vi "DynamixelConfigure.vi"() -> ()   [LabVIEW 2013]
doc: "Set the Dynamixels to the settings we want. Should only need to be run one per group of Dynamixels - they're supposed to remember their settings.\n\nElizabeth Mahon, 4-7-2014"
uses:
  <instrlib>/Dynamixel Motor/Public/Motor Operation/Low Level/Baud Setting.ctl
  <instrlib>/Dynamixel Motor/Dynamixel Motor.lvlib
panel:
  out "Found right # of motors?":bool
  in  "# of motors":i32=3
  in  "VISA resource name":refnum<visa-resource-name>
  # "SET THESE BEFORE RUNNING!"
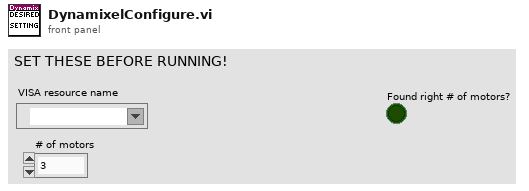
[diagram p1: front panel]
types:
  T1 = typedef "Dynamixel Motor.lvlib/Baud Setting.ctl" = u8
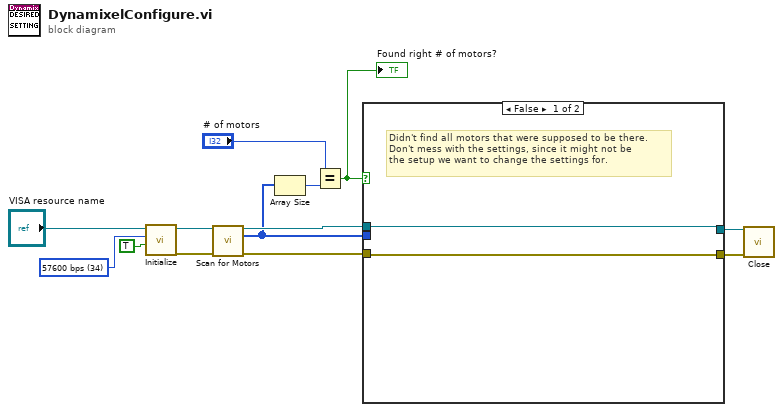
[diagram p0: block diagram]
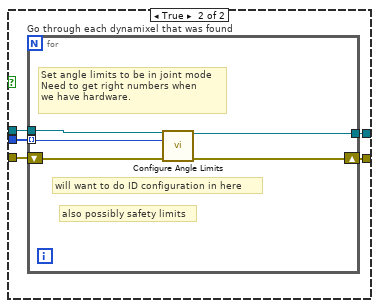
[diagram p2: hidden frame]
diagram:
  w12 = T1 34 items=["1,000,000 bps"=1, "500,000 bps"=3, "400,000 bps"=4, "250,000 bps"=7, "200,000 bps"=9, "115200 bps"=16, "57600 bps"=34, "19200 bps"=103, "9600 bps"=207] ("Baud rate (57600 bps)")
  n1 = call <instrlib>:"Initialize.vi"("Force Baud Rate (True)"=TRUE, "Baud rate (57600 bps)"=w12, "VISA resource name"="VISA resource name") -> ("error out"=w9:errorcluster, "VISA resource name out"=w10:refnum<visa-resource-name>)  [unwired: 7 in]
  n2 = call <instrlib>:"Scan for Motors.vi"("VISA resource name"=w10, "error in (no error)"=w9) -> ("VISA resource name out"=w8:refnum<visa-resource-name>, "Motors IDs Found"=w4:u8[], "error out"=w6:errorcluster)  [unwired: 11 in]
  n3 = Array Size(array=w4) -> (size(s)=w3:i32)
  n4 = Equal?(x="# of motors", y=w3) -> (x = y?=w1:bool)
  "Found right # of motors?" <- w1
  n5 = case shown="False" w1 {
    tunnel: w4 -> [_ w20]
    tunnel: w8 -> [w15 w19]
    tunnel: [w15 w18] -> w7
    tunnel: w6 -> [w14 w17]
    tunnel: [w14 w16] -> w5
    frame False {
      # "Didn't find all motors that were supposed to be there.\nDon't mess with the settings, since it might not be\nthe setup we want to change the settings for."
    }
    frame True {
      n6 = for "Go through each dynamixel that was found" {
        tunnel: w20 -> [w24] mode=indexing
        tunnel: w19 -> [w25]
        tunnel: [w23] -> w18
        shift-right: [w22] -> w16
        shift-left: w17 -> [w21]
        # "also possibly safety limits"
        # "will want to do ID configuration in here"
        # "Set angle limits to be in joint mode\nNeed to get right numbers when\nwe have hardware."
        n7 = call <instrlib>:"Configure Angle Limits.vi"("VISA resource name"=w25, "Motor ID (0)"=w24, "error in (no error)"=w21) -> ("VISA resource name out"=w23:refnum<visa-resource-name>, "error out"=w22:errorcluster)  [unwired: 11 in]
      }
    }
  }
  n8 = call <instrlib>:"Close.vi"("error in (no error)"=w5, "VISA resource name"=w7) -> ()  [unwired: 9 in, 1 out]
